vi "DAQ_Dig Freq Meas Initialize.vi"(0 "Physical Channel (counter)":tag, 2 "Input Terminal":tag, 7 "Global Channel (counter)":refnum<k21>, 11 "error in":errorcluster) -> (4 "DAQmx Task Out":refnum<k21>, 15 "error out":errorcluster)   [LabVIEW 2021, in "DAQ_Digital Frequency Measurement.lvlib"]
doc: "Initialize Counter Input task for digital frequency measurement.\n\nProvide either Physical channel or Global channel for counters to use.\nIf both physical and global channels are provided, Global Channels will take precedence\n\nNote: Multiple counters cannot be initialized in the same task for input operations. Use separate task for each counter."
uses:
  DAQ_Digital Frequency Measurement.lvlib
  <vilib>/DAQmx/create/channels.llb/DAQmx Create Channel (CI-Frequency).vi
  <resource>/objmgr/daqmx.rc
panel:
  # "Inputs"
  # "Outputs"
  # "Overview:\nThis VI initializes a counter input channel for digital frequency measurement and provides the DAQmx Task Out\n\nHardware Requirement: A compatible PXI, PCIe, USB, cDAQ or Testscale device\n\nSoftware Requirement: NI DAQmx 2022Q4 or later\n\nInstructions:\n1. Enter Input Terminal on which the signal to be measured. Refer Help for more details on the default terminals of each counters. User can configure different PFI lines as well. \n2. Enter counter which should be used for Digital Pattern Measurement has to be done in Physical Channel (counter) control. (Or) Enter Global channels to use it instead of initiating a new task. User must configure only one input. If both are provided, Global Channels will take precedence.\n3. Get the Digital frequency measurement task from DAQmx Task Out which stores the reference to the virtual counter input channel.\n\nNotes: \n1. User can use the DAQmx Task on other VI in this library to configure and initiate digital frequency measurement task.\n2. Multiple counters cannot be initialized in the same task for input operations. Use separate task for each counter."
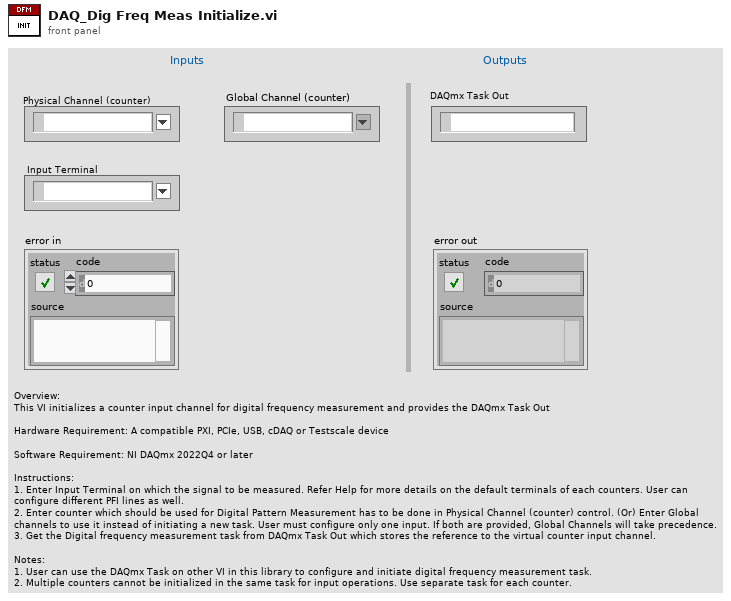
[diagram p1: front panel]
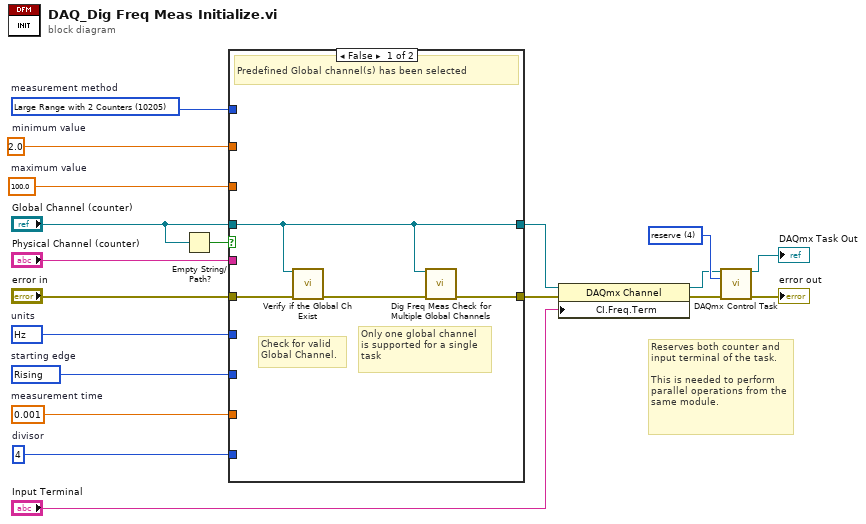
[diagram p0: block diagram]
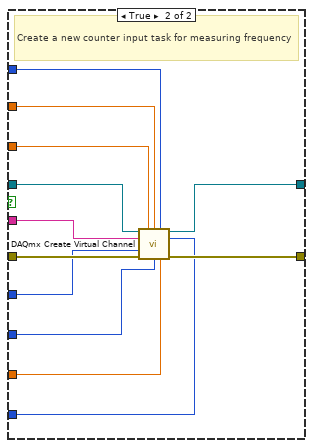
[diagram p2: hidden frame]
diagram:
  w8 = 4 items=["verify"=2, "reserve"=4, "commit"=3, "unreserve"=5, "abort"=6] ("action")
  w9 = u32 4  # divisor
  w10 = 0.001  # measurement time
  w11 = 10280 items=["Rising"=10280, "Falling"=10171]  # starting edge
  w12 = 2.0  # minimum value
  w13 = 100.0  # maximum value
  w14 = 10205 items=["Low Frequency with 1 Counter"=10105, "High Frequency with 2 Counters"=10157, "Large Range with 2 Counters"=10205, "Dynamic Averaging"=16065]  # measurement method
  w15 = 10373 items=["Hz"=10373, "Ticks"=10304, "From Custom Scale"=10065]  # units
  # "Reserves both counter and input terminal of the task.\n\nThis is needed to perform parallel operations from the same module."
  n1 = Empty String/Path?(string/path="Global Channel (counter)") -> (empty?=w17:bool)
  n2 = case shown="False" w17 {
    tunnel: "Physical Channel (counter)" -> [_ w25]
    tunnel: "Global Channel (counter)" -> [w21 w35]
    tunnel: "error in" -> [w23 w33]
    tunnel: [w22 w34] -> w5
    tunnel: w15 -> [_ w32]
    tunnel: w14 -> [_ w31]
    tunnel: w13 -> [_ w30]
    tunnel: w12 -> [_ w29]
    tunnel: w11 -> [_ w28]
    tunnel: w10 -> [_ w27]
    tunnel: w9 -> [_ w26]
    tunnel: [w21 w24] -> w3
    frame False {
      # "Only one global channel\nis supported for a single\ntask"
      # "Check for valid \nGlobal Channel."
      # "Predefined Global channel(s) has been selected"
      n3 = call "Verify if the Global Ch Exist.vi"("Global Channels"=w21, "error in (no error)"=w23) -> ("error out"=w20:errorcluster)  [unwired: 13 in]
      n4 = call "Dig Freq Meas Check for Multiple Global Channels.vi"("Global Channel In"=w21, "error in (no error)"=w20) -> ("error out"=w22:errorcluster)  [unwired: 12 in, 1 out]
    }
    frame True {
      # "Create a new counter input task for measuring frequency"
      n5 = call-poly <vilib>:"DAQmx Create Virtual Channel.vi"("task in"=w35, "maximum value"=w30, "minimum value"=w29, "measurement method"=w31, "counter"=w25, "divisor"=w26, "units"=w32, "error in"=w33, "starting edge"=w28, "measurement time"=w27) -> ("task out"=w24:refnum<k21>, "error out"=w34:errorcluster)  [unwired: 4 in]
    }
  }
  n6 = property class="DAQmx Channel"(reference=w3, error in=w5, "CI.Freq.Term"="Input Terminal") -> (reference out=w2:refnum<k21>, error out=w4:errorcluster)
  n7 = call <vilib>:"DAQmx Control Task.vi"("task/channels in"=w2, "action"=w8, "error in"=w4) -> ("task out"=→"DAQmx Task Out":refnum<k21>, "error out"=→"error out":errorcluster)  [unwired: 11 in]
